vi "002_Panel01.vi"(11 "Queue Ref In":T1={"UI"=refnum, "Message"=refnum, "Data"=refnum, "Caller"=refnum, "Name"="000 Common", "Data Path"=path "", "Class Path"=path "", "SubPanel"=refnum, "Project Name"="", "MNT"="", "Title"="", "Data Source"=refnum, "Queue List"={}, "VI"=refnum, "UE"=refnum}) -> ()   [LabVIEW 2020]
uses:
  Alin/QMH/000 Module Data Type.ctl
  Alin/QMH/Queue Message.ctl
  <vilib>/Utility/file.llb/Read Delimited Spreadsheet (string).vi
  <vilib>/Utility/file.llb/Write Delimited Spreadsheet (string).vi
panel:
  in  "PanelSelect_00":u16(ring)
  in  "PanelSelect_01":u16(ring)
  in  "Panel Config":bool
  in  "Panel Refresh":bool
  in  "PanelSelect_02":u16(ring)
  in  "PanelSelect_03":u16(ring)
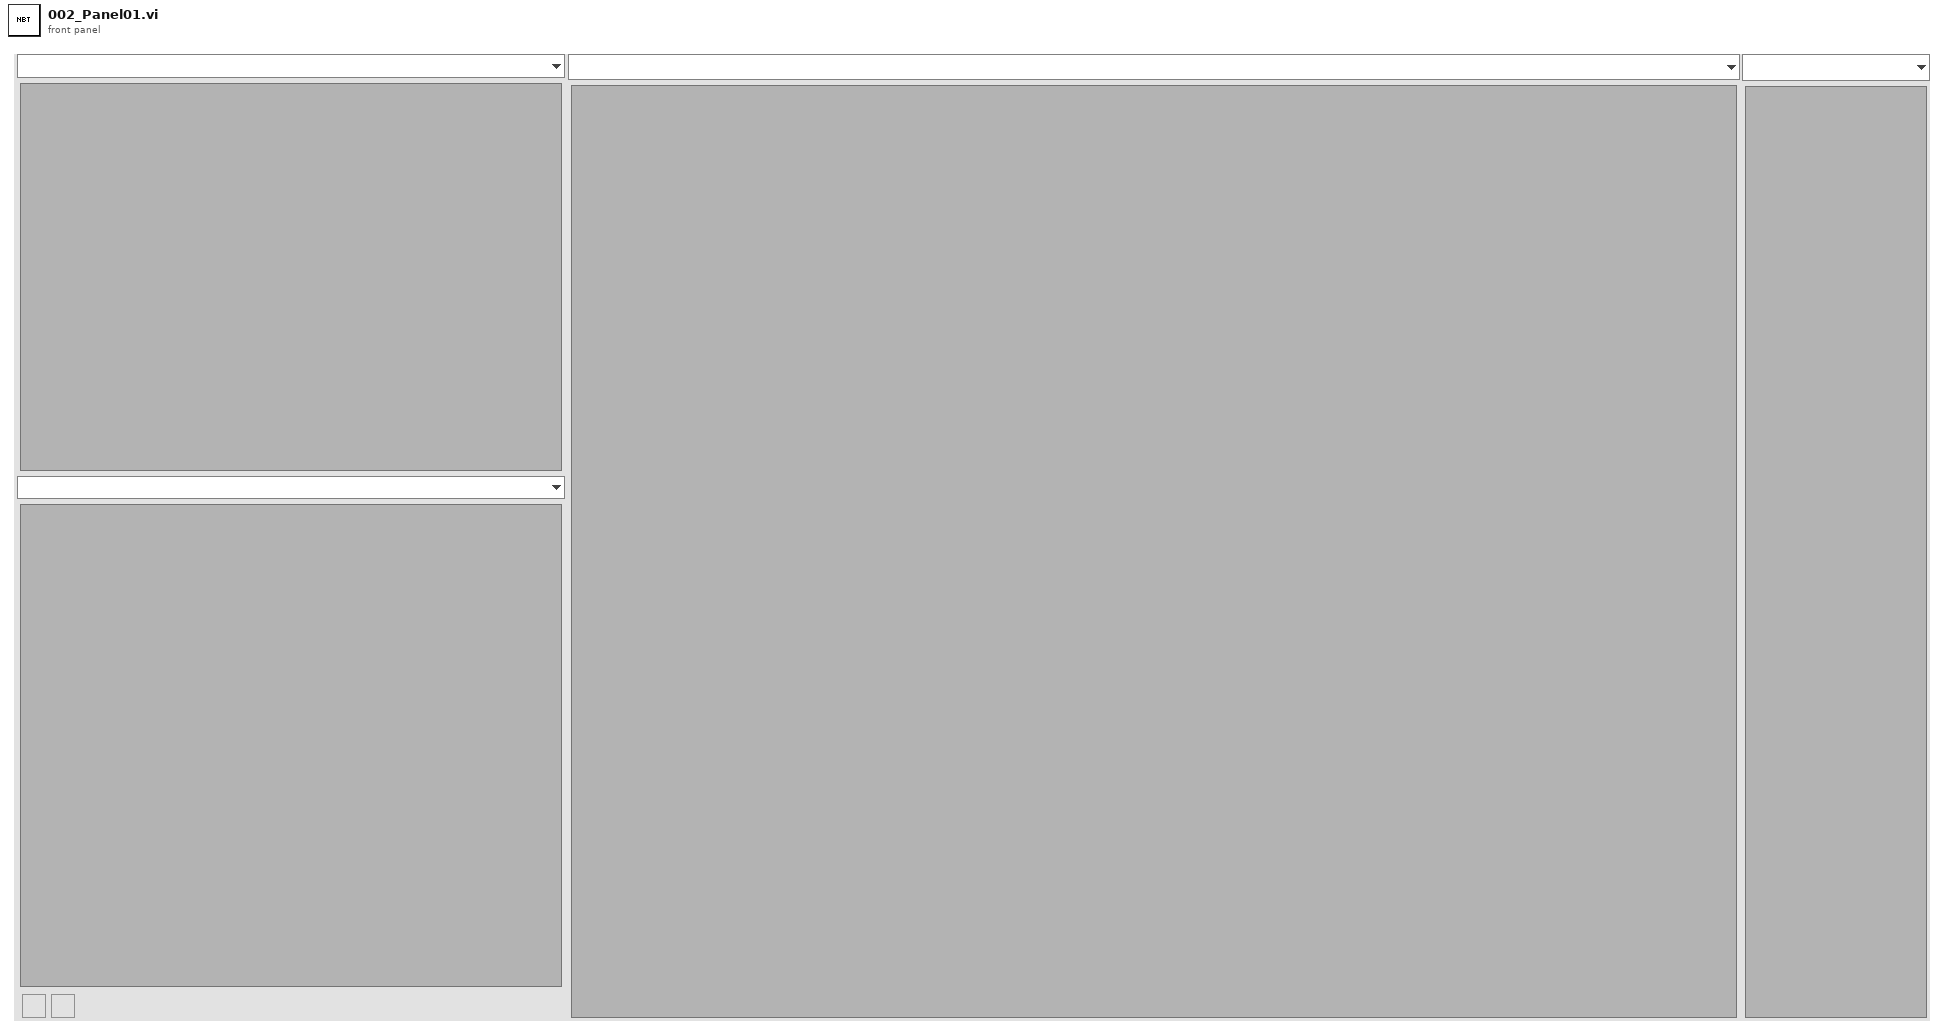
[diagram p1: front panel]
types:
  T1 = typedef "000 Module Data Type.ctl" = cluster{"UI":refnum<queue>, "Message":refnum<queue>, "Data":refnum<queue>, "Caller":refnum<queue>, "Name":string, "Data Path":path, "Class Path":path, "SubPanel":refnum<vi>, "Project Name":string, "MNT":string, "Title":string, "Data Source":refnum<queue>, "Queue List":map{string, refnum<queue>}, "VI":refnum<vi>, "UE":refnum<user-event>}
  T2 = typedef "eventvkey.ctl" = enum16{"ASCII", "Enter", "Return", "Shift", "Ctrl", "Alt", "Cmd", "Opt", "Caps", "NumLock", "Clear", "Break", "Up", "Down", "Left", "Right", "Insert", "Delete", "Home", "End", "PageUp", "PageDown", "Escape", "Help", "Pause", "ScrollLock", "F1", "F2", "F3", "F4", "F5", "F6", "F7", "F8", "F9", "F10", "F11", "F12", "F13", "F14", "F15", "F16", "F17", "F18", "F19", "F20", "F21", "F22", "F23", "F24", "Play", "VolumeUp", "VolumeDown", "Mute", "Two Byte Char"}
  T3 = cluster{"Shift":bool, "Ctrl":bool, "Alt":bool, "Cmd":bool, "Opt":bool}
  T4 = cluster{"Queue":T1, "SubPanel":cluster{"SubPanel01":refnum<vi>, "SubPanel02":refnum<vi>, "SubPanel03":refnum<vi>, "SubPanel04":refnum<vi>}, "Panel Name":string[], "PanelSelect":cluster{"PanelSelect_00":refnum<vi>, "PanelSelect_01":refnum<vi>, "PanelSelect_02":refnum<vi>, "PanelSelect_03":refnum<vi>}, "Panel Index":string[]}
  T5 = cluster{"SubPanel01":refnum<vi>, "SubPanel02":refnum<vi>, "SubPanel03":refnum<vi>, "SubPanel04":refnum<vi>}
  T6 = cluster{"PanelSelect_00":refnum<vi>, "PanelSelect_01":refnum<vi>, "PanelSelect_02":refnum<vi>, "PanelSelect_03":refnum<vi>}
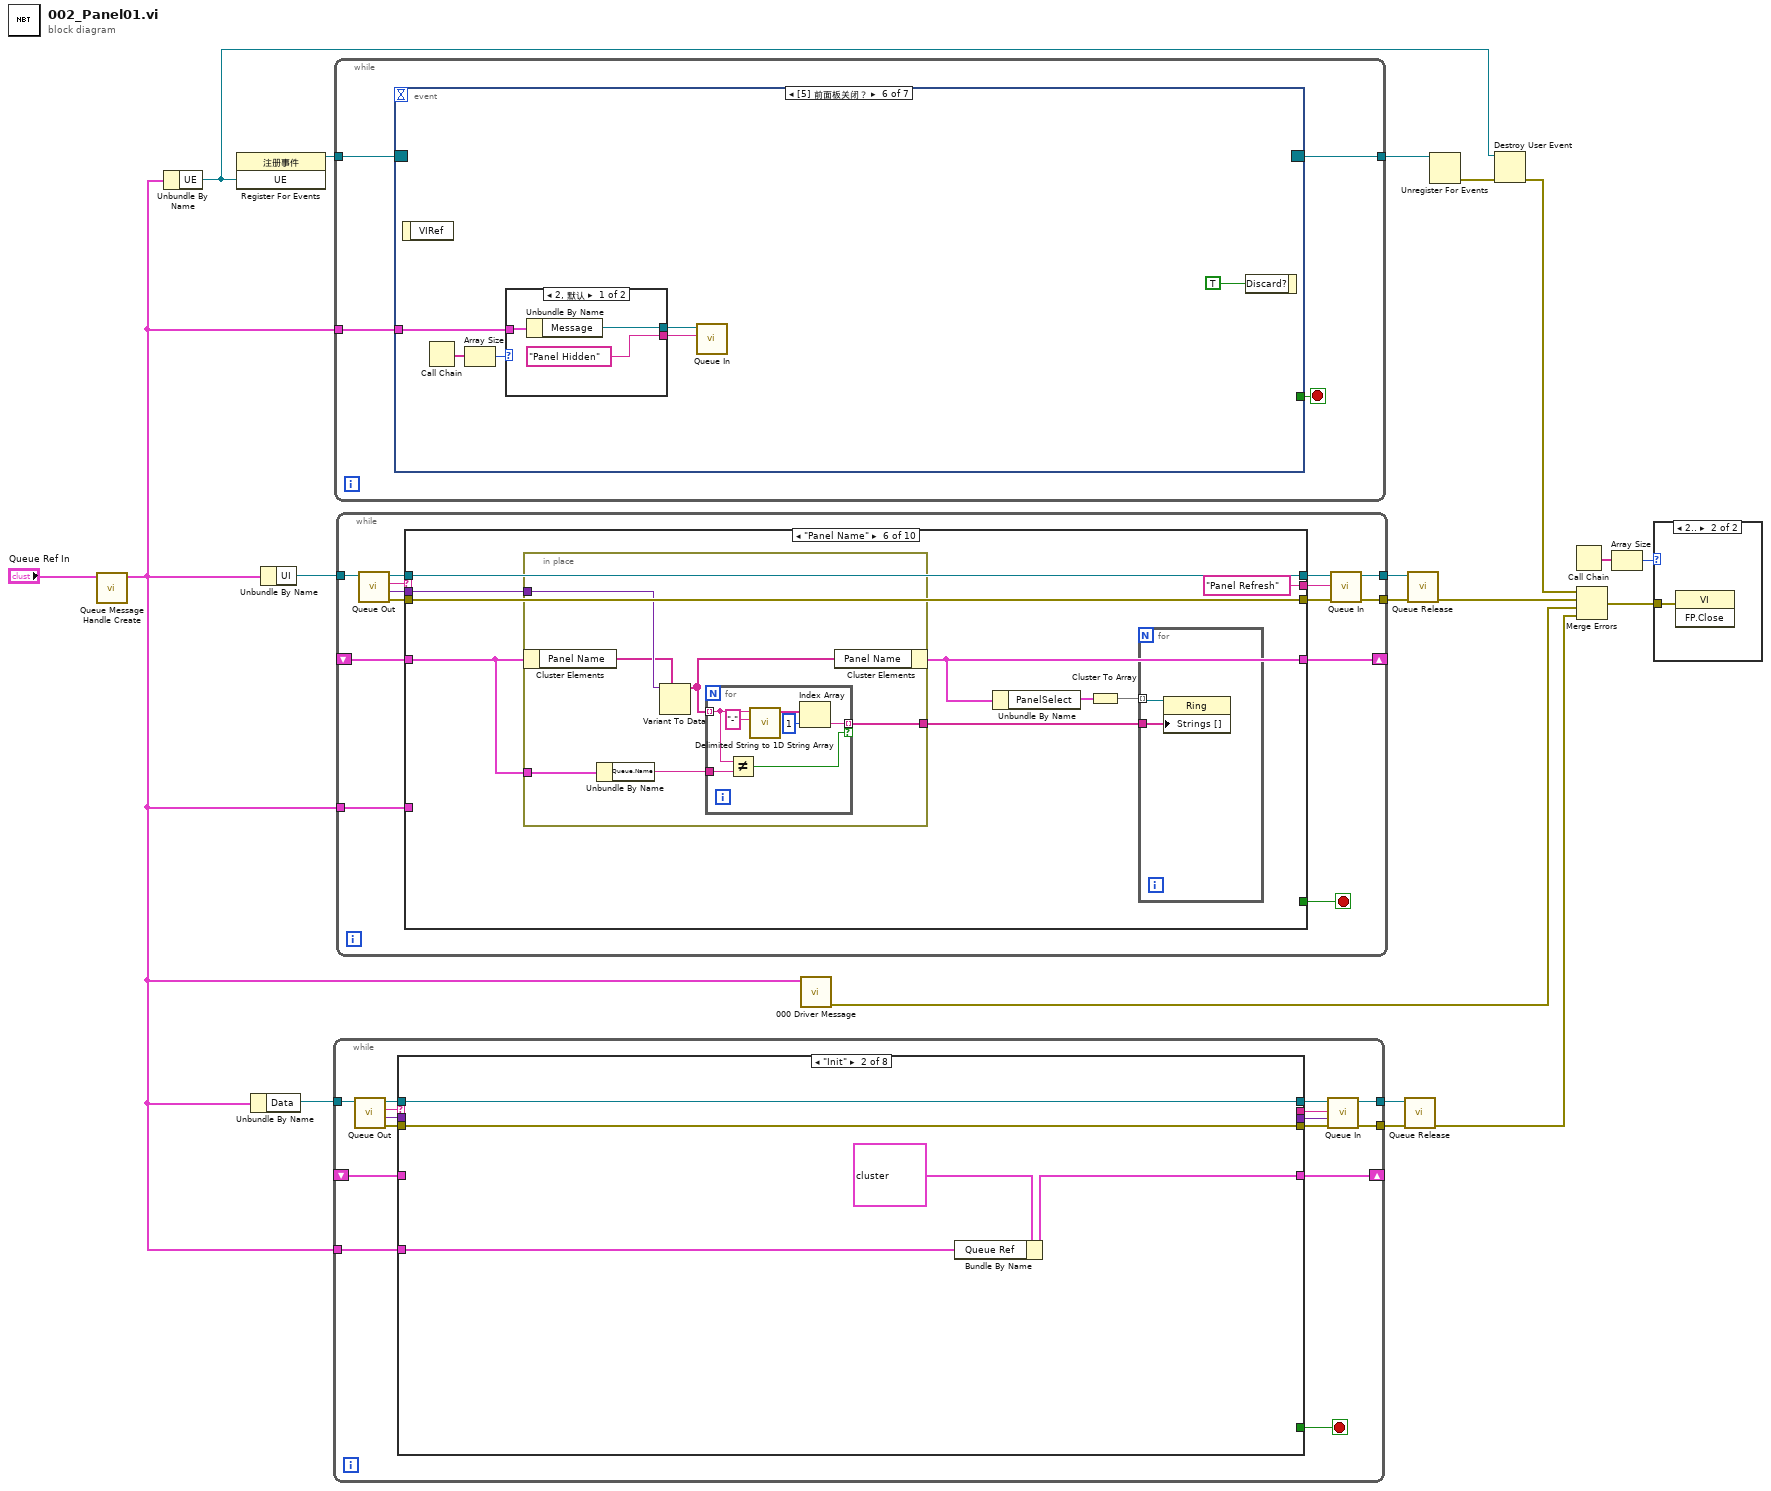
[diagram p0: block diagram]
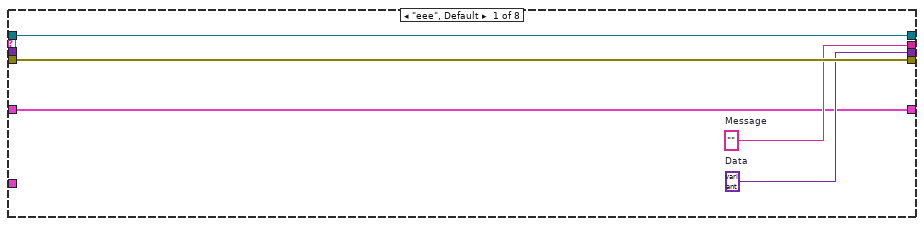
[diagram p2: hidden frame]
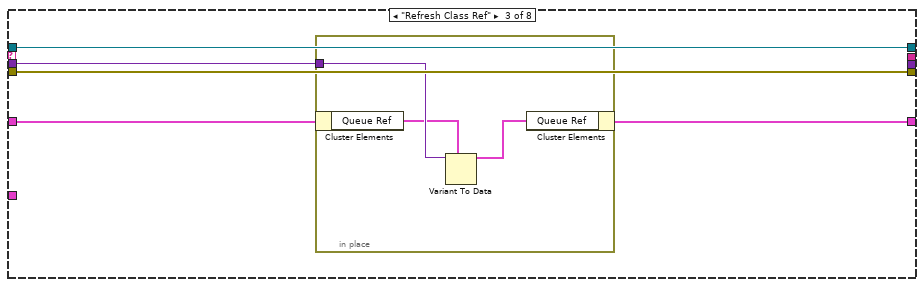
[diagram p3: hidden frame]
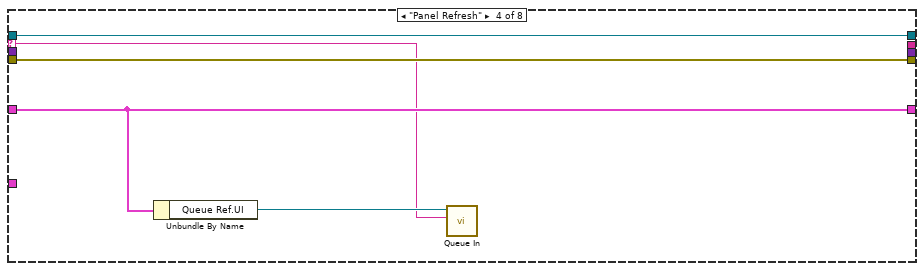
[diagram p4: hidden frame]
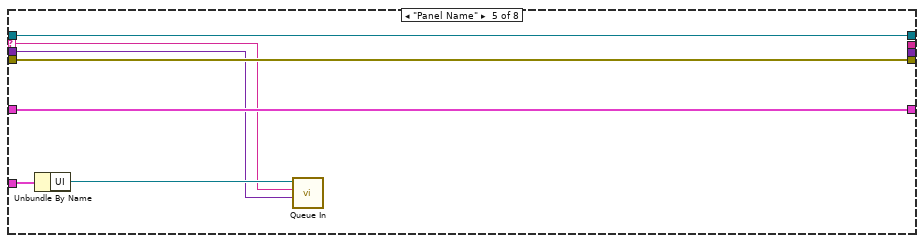
[diagram p5: hidden frame]
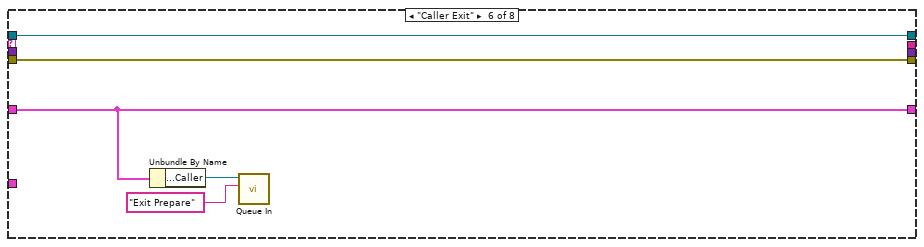
[diagram p6: hidden frame]
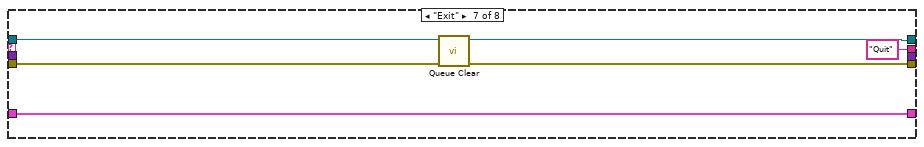
[diagram p7: hidden frame]
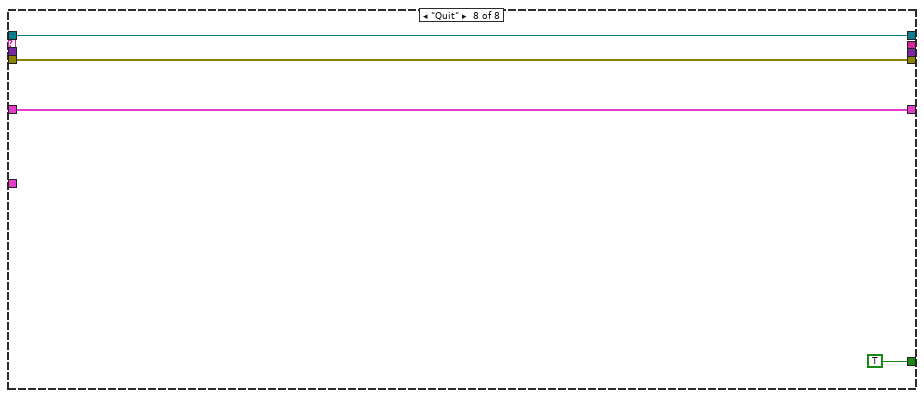
[diagram p8: hidden frame]
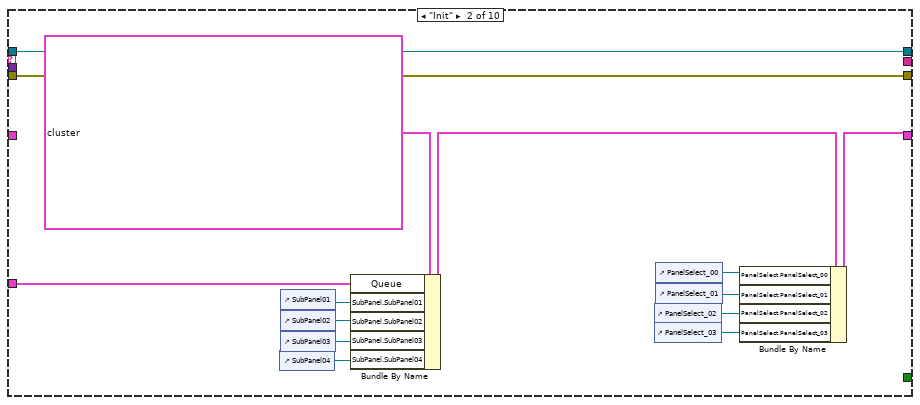
[diagram p11: hidden frame]
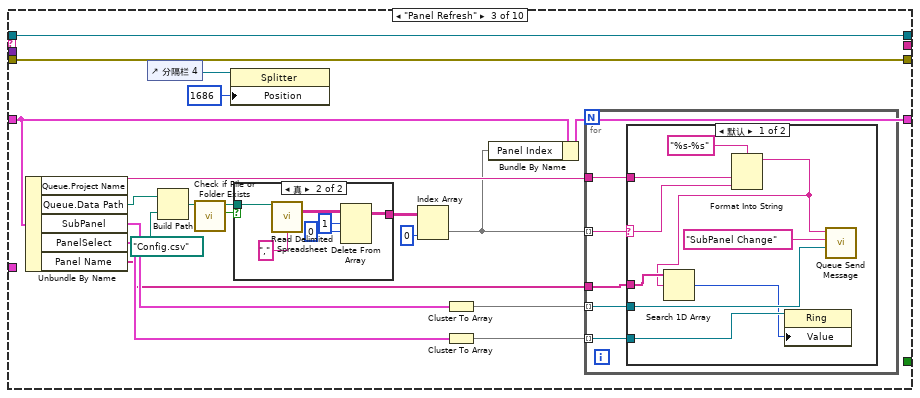
[diagram p12: hidden frame]
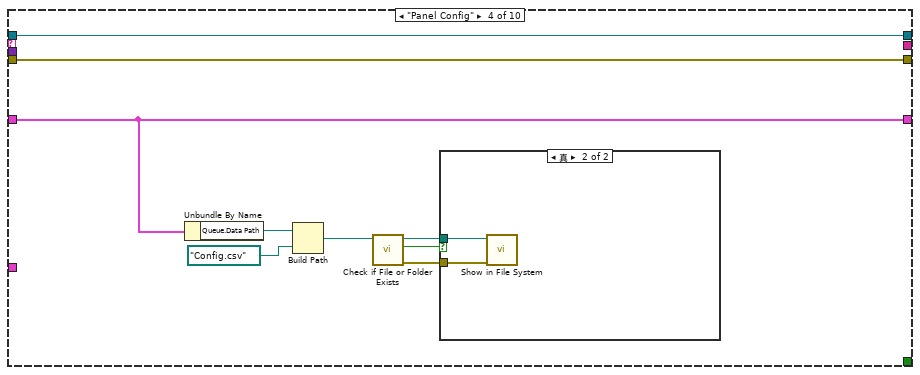
[diagram p15: hidden frame]
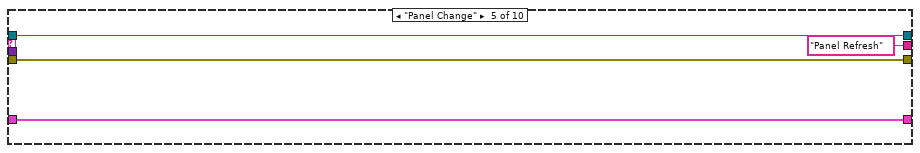
[diagram p17: hidden frame]
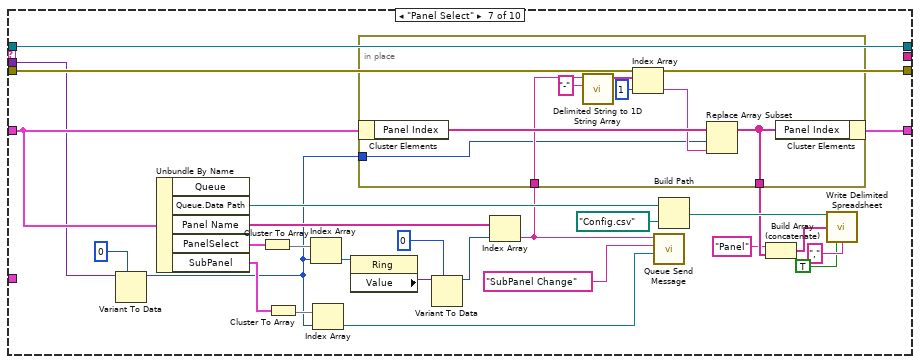
[diagram p18: hidden frame]
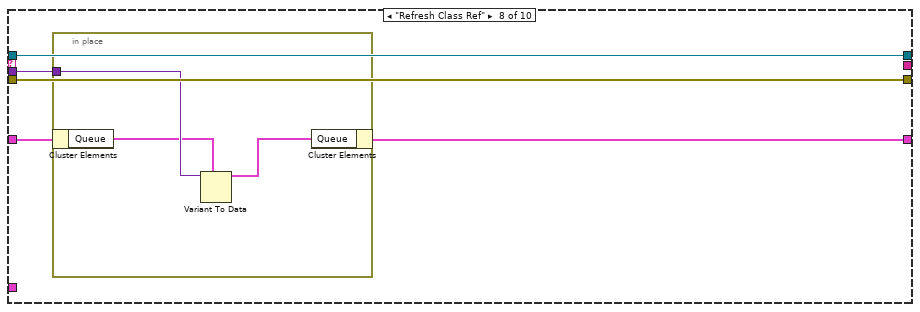
[diagram p19: hidden frame]
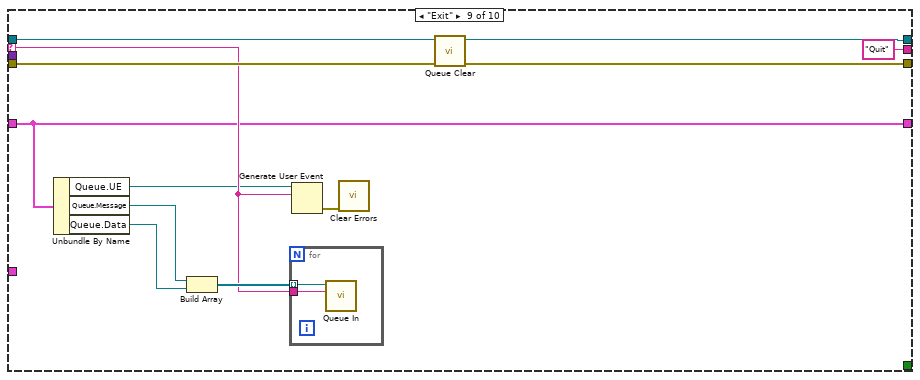
[diagram p20: hidden frame]
diagram:
  n1 = call "Queue Message Handle Create.vi"("Queue Ref In"="Queue Ref In") -> ("Queue Ref Out"=w1:T1)  [unwired: 9 in, 1 out]
  n2 = Unbundle By Name(w1) -> ("UE"=w2:refnum<user-event>)
  n3 = register-events(w2) -> (reference out=w3:refnum<event-registration>)  [unwired: 2 in, 1 out]
  n4 = Unbundle By Name(w1) -> ("Data"=w16:refnum<queue>)
  n5 = Unbundle By Name(w1) -> ("UI"=w8:refnum<queue>)
  n6 = while {
    tunnel: w16 -> [w30]
    tunnel: [w27] -> w14
    tunnel: [w26] -> w15
    shift-right: [w22] -> _
    shift-left: _ -> [w21]
    tunnel: w1 -> [w20]
    stop <- w34 stop-if-true
    n7 = call "Queue Out.vi"("Queue In"=w30) -> ("error out"=w33:errorcluster, "Data"=w31:variant, "Message"=w32:string, "Queue Out"=w29:refnum<queue>)  [unwired: 6 in, 1 out]
    n8 = case shown="\"Init\"" w32 {
      selector: w32 -> [_ _ _ w53 w59 _ _ _]
      tunnel: w29 -> [w39 w44 w49 w57 w64 w69 w74 w78]
      tunnel: w33 -> [w38 w43 w48 w56 w63 w68 w72 w79]
      tunnel: [w39 w44 w49 w57 w64 w69 w73 w78] -> w28
      tunnel: [w38 w43 w48 w56 w63 w68 w71 w79] -> w25
      tunnel: [w37 _ _ _ _ _ "Quit" _] -> w24
      tunnel: [_ _ _ _ _ _ _ TRUE] -> w34
      tunnel: [w36 _ _ _ _ _ _ _] -> w23
      tunnel: w31 -> [_ _ w45 _ w58 _ _ _]
      tunnel: [w35 w41 w46 w55 w62 w67 w70 w76] -> w22
      tunnel: w21 -> [w35 _ w47 w55 w62 w67 w70 w76]
      tunnel: w20 -> [_ w40 _ _ w61 _ _ _]
      frame "eee", Default {
        w36 = variant  # Data
        w37 = ""  # Message
      }
      frame "Init" {
        n9 = Bundle By Name(cluster=cluster{"Queue Ref ":T1} {"Queue Ref "={"UI"=refnum, "Message"=refnum, "Data"=refnum, "Caller"=refnum, "Name"="000 Common", "Data Path"=path "", "Class Path"=path "", "SubPanel"=refnum, "Project Name"="", "MNT"="", "Title"="", "Data Source"=refnum, "Queue List"={}, "VI"=refnum, "UE"=refnum}}, "Queue Ref"=w40) -> (w41:cluster{"Queue Ref ":T1})
      }
      frame "Refresh Class Ref" {
        n10 = in-place {
          in-place-border: w45 -> [w52]
          n11 = in-place-cluster #1(w47) -> ("Queue Ref"=w51:T1)
          n12 = Variant To Data(type=w51, Variant=w52) -> (data=w50:T1)  [unwired: 1 in, 1 out]
          n13 = in-place-cluster #1("Queue Ref"=w50) -> (w46:cluster{"Queue Ref ":T1})
        }
      }
      frame "Panel Refresh" {
        n14 = Unbundle By Name(w55) -> ("Queue Ref.UI"=w54:refnum<queue>)
        n15 = call "Queue In.vi"("Message"=w53, "Queue In"=w54) -> ()  [unwired: 8 in, 2 out]
      }
      frame "Panel Name" {
        n16 = Unbundle By Name(w61) -> ("UI"=w60:refnum<queue>)
        n17 = call "Queue In.vi"("Data"=w58, "Message"=w59, "Queue In"=w60) -> ()  [unwired: 7 in, 2 out]
      }
      frame "Caller Exit" {
        n18 = Unbundle By Name(w67) -> ("Queue Ref.Caller"=w66:refnum<queue>)
        n19 = call "Queue In.vi"("Message"="Exit Prepare", "Queue In"=w66) -> ()  [unwired: 8 in, 2 out]
      }
      frame "Exit" {
        n20 = call "Queue Clear.vi"("error in (no error)"=w72, "Queue In"=w74) -> ("error out"=w71:errorcluster, "Queue Out"=w73:refnum<queue>)  [unwired: 8 in]
      }
      frame "Quit" {
      }
    }
    n21 = call "Queue In.vi"("error in (no error)"=w25, "Data"=w23, "Message"=w24, "Queue In"=w28) -> ("error out"=w26:errorcluster, "Queue Out"=w27:refnum<queue>)  [unwired: 6 in]
  }
  n22 = while {
    tunnel: w3 -> [w83]
    tunnel: [w81] -> w4
    tunnel: w1 -> [w80]
    stop <- w82 stop-if-true
    n23 = event shown="[5] 前面板关闭？" {
      selector: w83 -> [_ _ _ _ _ _ _]
      dyn-events: [_ _ _ _ _ _ _] -> w81
      timeout: _ -> [_ _ _ _ _ _ _]
      tunnel: [_ _ _ _ w96 _ _] -> w82
      tunnel: w80 -> [_ w87 w91 w95 _ w99 w121]
      event Timeout {
        n24 = event-data() -> ()  [unwired: 1 in, 1 out]
      }
      event "Panel Refresh", "Panel Config": Value Change {
        n25 = event-data() -> ("CtlRef"=w85:refnum<vi>)  [unwired: 1 in]
        n26 = Unbundle By Name(w87) -> ("UI"=w86:refnum<queue>)
        n27 = property class="Bool"(reference=w85) -> ("Label.Text"=w84:string)  [unwired: 1 in, 2 out]
        n28 = call "Queue In.vi"("Message"=w84, "Queue In"=w86) -> ()  [unwired: 8 in, 2 out]
      }
      event Key Down {
        n29 = event-data() -> ("Char"=w92:i16, "VKey"=w90:T2, "Mods"=w89:cluster{"Num Pad":bool, "Menu Key":bool}, "PlatMods"=w88:T3)  [unwired: 1 in]
        n30 = call "Queue Key Down.vi"("Queue Ref Out"=w91, "C"=w92, "Platform Key"=w88, "Group Key"=w89, "V Key"=w90) -> ()  [unwired: 6 in, 1 out]
      }
      event Panel Resize; Pane Size {
        n31 = event-data() -> ()  [unwired: 1 in, 2 out]
        n32 = Unbundle By Name(w95) -> ("Data"=w94:refnum<queue>)
        n33 = call "Queue In.vi"("Message"="Panel Adjust", "Queue In"=w94) -> ()  [unwired: 8 in, 2 out]
      }
      event User Event {
        n34 = event-data() -> ("Message"=w98:string)  [unwired: 1 in]
        n35 = Equal?(x=w98, y="Exit") -> (x = y?=w96:bool)
      }
      event Panel Close? {
        n36 = event-data() -> ()  [unwired: 1 in, 1 out]
        n37 = Call Chain() -> (call chain=w103:string[])
        n38 = Array Size(array=w103) -> (size(s)=w102:i32)
        n39 = case shown="2, 默认" w102 {
          tunnel: w99 -> [w107 w110]
          tunnel: [w106 w109] -> w101
          tunnel: ["Panel Hidden" ("Message") "Exit Prepare" ("Message")] -> w100
          frame 2, Default {
            n40 = Unbundle By Name(w107) -> ("Message"=w106:refnum<queue>)
          }
          frame 1 {
            n41 = Unbundle By Name(w110) -> ("Message"=w109:refnum<queue>)
          }
        }
        n42 = call "Queue In.vi"("Message"=w100, "Queue In"=w101) -> ()  [unwired: 8 in, 2 out]
        n43 = event-data("Discard?"=TRUE ("放弃？")) -> ()  [unwired: 1 in, 1 out]
      }
      event "PanelSelect_01", "PanelSelect_00", "PanelSelect_02", "PanelSelect_03": Value Change {
        n44 = event-data() -> ("CtlRef"=w118:refnum<vi>)  [unwired: 1 in]
        n45 = Unbundle By Name(w121) -> ("UI"=w120:refnum<queue>)
        n46 = property class="Ring (严格)"(reference=w118) -> ("Label.Text"=w117:string)  [unwired: 1 in, 2 out]
        n47 = call <vilib>:"Delimited String to 1D String Array.vi"("delimiter"="_", "delimited string"=w117) -> ("string array"=w115:string[])  [unwired: 9 in]
        n48 = Index Array(array=w115, index=1 ("索引")) -> (element=w113:string)
        n49 = Fract/Exp String To Number(string=w113, default (0 dbl)=u32 0 ("默认(0 DBL)")) -> (number=w111:u32)  [unwired: 2 in, 1 out]
        n50 = call "Queue In.vi"("Data"=w111, "Message"="Panel Select", "Queue In"=w120) -> ()  [unwired: 7 in, 2 out]
      }
    }
  }
  n51 = while {
    tunnel: w8 -> [w131]
    tunnel: [w128] -> w6
    tunnel: [w127] -> w7
    shift-right: [w124] -> _
    shift-left: _ -> [w123]
    tunnel: w1 -> [w122]
    stop <- w135 stop-if-true
    n52 = call "Queue Out.vi"("Queue In"=w131) -> ("error out"=w134:errorcluster, "Data"=w132:variant, "Message"=w133:string, "Queue Out"=w130:refnum<queue>)  [unwired: 6 in, 1 out]
    n53 = case shown="\"Panel Name\"" w133 {
      selector: w133 -> [_ _ _ _ _ _ _ _ w280 _]
      tunnel: w130 -> [w138 w152 w172 w201 w207 w216 w258 w271 w285 w291]
      tunnel: w134 -> [w137 w151 w171 w200 w206 w215 w257 w270 w283 w292]
      tunnel: [w138 w152 w172 w201 w207 w216 w258 w271 w284 w291] -> w129
      tunnel: [w137 w151 w171 w200 w206 w215 w257 w270 w282 w292] -> w126
      tunnel: [_ _ _ _ "Panel Refresh" "Panel Refresh" _ _ "Quit" _] -> w125
      tunnel: [_ _ _ _ _ _ _ _ _ TRUE] -> w135
      tunnel: w132 -> [_ _ _ _ _ w214 w253 w268 _ _]
      tunnel: [w136 w143 w157 w198 w205 w213 w240 w267 w278 w289] -> w124
      tunnel: w123 -> [w136 _ w170 w198 w205 w208 w256 w269 w278 w289]
      tunnel: w122 -> [_ w148 _ _ _ _ _ _ _ _]
      frame "eee", Default {
      }
      frame "Init" {
        n54 = control-ref of="SubPanel04"() -> (w144:refnum<vi>)
        n55 = control-ref of="SubPanel01"() -> (w145:refnum<vi>)
        n56 = control-ref of="SubPanel02"() -> (w146:refnum<vi>)
        n57 = control-ref of="SubPanel03"() -> (w147:refnum<vi>)
        n58 = Bundle By Name(cluster=T4 {"Queue"={"UI"=refnum, "Message"=refnum, "Data"=refnum, "Caller"=refnum, "Name"="000 Common", "Data Path"=path "", "Class Path"=path "", "SubPanel"=refnum, "Project Name"="", "MNT"="", "Title"="", "Data Source"=refnum, "Queue List"={}, "VI"=refnum, "UE"=refnum}, "SubPanel"={"SubPanel01"=refnum, "SubPanel02"=refnum, "SubPanel03"=refnum, "SubPanel04"=refnum}, "Panel Name"=[], "PanelSelect"={"PanelSelect_00"=refnum, "PanelSelect_01"=refnum, "PanelSelect_02"=refnum, "PanelSelect_03"=refnum}, "Panel Index"=[]}, "Queue"=w148, "SubPanel.SubPanel01"=w145, "SubPanel.SubPanel02"=w146, "SubPanel.SubPanel03"=w147, "SubPanel.SubPanel04"=w144) -> (w149:T4)
        n59 = control-ref of="PanelSelect_02"() -> (w142:refnum<vi>)
        n60 = control-ref of="PanelSelect_03"() -> (w141:refnum<vi>)
        n61 = control-ref of="PanelSelect_00"() -> (w139:refnum<vi>)
        n62 = control-ref of="PanelSelect_01"() -> (w140:refnum<vi>)
        n63 = Bundle By Name(cluster=w149, "PanelSelect.PanelSelect_00"=w139, "PanelSelect.PanelSelect_01"=w140, "PanelSelect.PanelSelect_02"=w142, "PanelSelect.PanelSelect_03"=w141) -> (w143:T4)
      }
      frame "Panel Refresh" {
        n64 = Unbundle By Name(w170) -> ("Queue.Project Name"=w160:string, "Queue.Data Path"=w163:path, "SubPanel"=w165:T5, "PanelSelect"=w155:T6, "Panel Name"=w153:string[])
        n65 = control-ref of="分隔栏 4"() -> (w159:refnum<vi>)
        n66 = Build Path(base path=w163, name or relative path=path "Config.csv" ("名称或相对路径")) -> (appended path=w161:path)
        n67 = call <vilib>:"Check if File or Folder Exists.vi"("path"=w161) -> ("file or folder exists?"=w168:bool, "dup path"=w169:path)  [unwired: 8 in, 1 out]
        n68 = property class="Splitter"(reference=w159, "Position"=1686 ("分隔栏位置")) -> ()  [unwired: 1 in, 2 out]
        n69 = case shown="真" w168 {
          tunnel: w169 -> [_ w191]
          tunnel: [_ w187] -> w167
          frame False {
          }
          frame True {
            n70 = call-poly <vilib>:"Read Delimited Spreadsheet.vi"("file path (dialog if empty)"=w191, "delimiter (\\t)"="," ("delimiter (\\t)")) -> ("all rows"=w190:string[][])  [unwired: 8 in, 5 out]
            n71 = Delete From Array(array=w190, length=1 ("长度"), index (row)=0 ("索引 (行)")) -> (array with subset deleted=w187:string[][])  [unwired: 1 in, 1 out]
          }
        }
        n72 = Index Array(array=w167, index (col)=0 ("禁用的索引 (列)")) -> (element=w156:string[])  [unwired: 1 in]
        n73 = Cluster To Array(cluster=w165) -> (array=w164:refnum<vi>[])
        n74 = Cluster To Array(cluster=w155) -> (array=w154:refnum<vi>[])
        n75 = Bundle By Name(cluster=w170, "Panel Index"=w156) -> (w157:T4)
        n76 = for {
          tunnel: w156 -> [w175] mode=indexing
          tunnel: w164 -> [w177] mode=indexing
          tunnel: w160 -> [w176]
          tunnel: w154 -> [w174] mode=indexing
          tunnel: w153 -> [w173]
          n77 = case shown="默认" w175 {
            selector: w175 -> [w183 _]
            tunnel: w177 -> [w185 _]
            tunnel: w176 -> [w180 _]
            tunnel: w174 -> [w182 _]
            tunnel: w173 -> [w181 _]
            frame Default {
              n78 = Format Into String(format string="%s-%s" ("格式字符串"), w180, w183) -> (resulting string=w178:string)  [unwired: 2 in, 1 out]
              n79 = Search 1D Array(1D array=w181, element=w178) -> (index of element=w179:i32)  [unwired: 1 in]
              n80 = property class="Ring"(reference=w182, "Value"=w179) -> ()  [unwired: 1 in, 2 out]
              n81 = call "Queue Send Message.vi"("Data"=w185, "Message"="SubPanel Change", "Queue Name"=w178) -> ()  [unwired: 6 in, 3 out]
            }
            frame "" {
            }
          }
        }
      }
      frame "Panel Config" {
        n82 = Unbundle By Name(w198) -> ("Queue.Data Path"=w197:path)
        n83 = Build Path(base path=w197, name or relative path=path "Config.csv" ("名称或相对路径")) -> (appended path=w196:path)
        n84 = call <vilib>:"Check if File or Folder Exists.vi"("path"=w196) -> ("error out"=w193:errorcluster, "file or folder exists?"=w195:bool, "dup path"=w194:path)  [unwired: 8 in]
        n85 = case shown="真" w195 {
          tunnel: w194 -> [_ w203]
          tunnel: w193 -> [_ w202]
          frame False {
          }
          frame True {
            n86 = call <vilib>:"Show in File System.vi"("error in (no error)"=w202, "file or directory path"=w203) -> ()  [unwired: 9 in, 1 out]
          }
        }
      }
      frame "Panel Change" {
      }
      frame "Panel Name" {
        n87 = in-place {
          in-place-border: w214 -> [w224]
          in-place-border: [w221] -> w210
          in-place-border: w208 -> [w220]
          n88 = in-place-cluster #2(w208) -> ("Panel Name"=w223:string[])
          n89 = Unbundle By Name(w220) -> ("Queue.Name"=w219:string)
          n90 = Variant To Data(type=w223, Variant=w224) -> (data=w222:string[])  [unwired: 1 in, 1 out]
          n91 = for {
            tunnel: w222 -> [w227] mode=indexing
            tunnel: [w228] -> w221 mode=indexing if=w225
            tunnel: w219 -> [w226]
            n92 = Not Equal?(x=w227, y=w226) -> (x != y?=w225:bool)
            n93 = call <vilib>:"Delimited String to 1D String Array.vi"("delimiter"="-", "delimited string"=w227) -> ("string array"=w230:string[])  [unwired: 9 in]
            n94 = Index Array(array=w230, index=1 ("索引")) -> (element=w228:string)
          }
          n95 = in-place-cluster #2("Panel Name"=w222) -> (w213:T4)
        }
        n96 = Unbundle By Name(w213) -> ("PanelSelect"=w212:T6)
        n97 = Cluster To Array(cluster=w212) -> (array=w211:refnum<vi>[])
        n98 = for {
          tunnel: w211 -> [w218] mode=indexing
          tunnel: w210 -> [w217]
          n99 = property class="Ring"(reference=w218, "Strings []"=w217) -> ()  [unwired: 1 in, 2 out]
        }
      }
      frame "Panel Select" {
        n100 = Variant To Data(type=u32 0 ("数字"), Variant=w253) -> (data=w232:u32)  [unwired: 1 in, 1 out]
        n101 = Unbundle By Name(w256) -> ("Queue.Data Path"=w243:path, "Panel Name"=w255:string[], "PanelSelect"=w251:T6, "SubPanel"=w245:T5)  [unwired: 1 out]
        n102 = Cluster To Array(cluster=w251) -> (array=w250:refnum<vi>[])
        n103 = Cluster To Array(cluster=w245) -> (array=w246:refnum<vi>[])
        n104 = Index Array(array=w250, index=w232) -> (element=w249:refnum<vi>)
        n105 = Index Array(array=w246, index=w232) -> (element=w244:refnum<vi>)
        n106 = property class="Ring"(reference=w249) -> ("Value"=w248:variant)  [unwired: 1 in, 2 out]
        n107 = Variant To Data(type=u16 0 ("PanelSelect_03"), Variant=w248) -> (data=w239:u16)  [unwired: 1 in, 1 out]
        n108 = Index Array(array=w255, index=w239) -> (element=w238:string)
        n109 = in-place {
          in-place-border: w238 -> [w262]
          in-place-border: [w260] -> w236
          in-place-border: w232 -> [w259]
          n110 = in-place-cluster #3(w256) -> ("Panel Index"=w266:string[])
          n111 = call <vilib>:"Delimited String to 1D String Array.vi"("delimiter"="-", "delimited string"=w262) -> ("string array"=w264:string[])  [unwired: 9 in]
          n112 = Index Array(array=w264, index=1 ("索引")) -> (element=w261:string)
          n113 = Replace Array Subset(array=w266, new element=w261, index=w259) -> (w260:string[])
          n114 = in-place-cluster #3("Panel Index"=w260) -> (w240:T4)
        }
        n115 = call "Queue Send Message.vi"("Data"=w244, "Message"="SubPanel Change", "Queue Name"=w238) -> ()  [unwired: 6 in, 3 out]
        n116 = Build Path(base path=w243, name or relative path=path "Config.csv" ("名称或相对路径")) -> (appended path=w241:path)
        n117 = Build Array (concatenate)("Panel", w236) -> (w235:string[])
        n118 = call-poly <vilib>:"Write Delimited Spreadsheet.vi"("file path (dialog if empty)"=w241, "1D data"=w235, "transpose? (no:F)"=TRUE, "delimiter (\\t)"="," ("delimiter (\\t)")) -> ()  [unwired: 10 in, 2 out]
      }
      frame "Refresh Class Ref" {
        n119 = in-place {
          in-place-border: w268 -> [w274]
          n120 = in-place-cluster #4(w269) -> ("Queue"=w273:T1)
          n121 = Variant To Data(type=w273, Variant=w274) -> (data=w272:T1)  [unwired: 1 in, 1 out]
          n122 = in-place-cluster #4("Queue"=w272) -> (w267:T4)
        }
      }
      frame "Exit" {
        n123 = Unbundle By Name(w278) -> ("Queue.UE"=w277:refnum<user-event>, "Queue.Message"=w276:refnum<queue>, "Queue.Data"=w275:refnum<queue>)
        n124 = Build Array(w276, w275) -> (w281:refnum<queue>[])
        n125 = for {
          tunnel: w281 -> [w288] mode=indexing
          tunnel: w280 -> [w287]
          n126 = call "Queue In.vi"("Message"=w287, "Queue In"=w288) -> ()  [unwired: 8 in, 2 out]
        }
        n127 = Generate User Event(user event=w277, event data cluster=w280) -> (error out=w279:errorcluster)  [unwired: 2 in, 1 out]
        n128 = call <vilib>:"Clear Errors.vi"("error in (no error)"=w279) -> ()  [unwired: 5 in, 2 out]
        n129 = call "Queue Clear.vi"("error in (no error)"=w283, "Queue In"=w285) -> ("error out"=w282:errorcluster, "Queue Out"=w284:refnum<queue>)  [unwired: 8 in]
      }
      frame "Quit" {
      }
    }
    n130 = call "Queue In.vi"("error in (no error)"=w126, "Message"=w125, "Queue In"=w129) -> ("error out"=w127:errorcluster, "Queue Out"=w128:refnum<queue>)  [unwired: 7 in]
  }
  n131 = call "000 Driver Message.vi"("Queue In"=w1) -> ("error out"=w18:errorcluster)  [unwired: 8 in, 2 out]
  n132 = call "Queue Release.vi"("error in (no error)"=w15, "Queue In"=w14) -> ("error out"=w17:errorcluster)  [unwired: 9 in]
  n133 = call "Queue Release.vi"("error in (no error)"=w7, "Queue In"=w6) -> ("error out"=w10:errorcluster)  [unwired: 9 in]
  n134 = Unregister For Events(event registration refnum=w4) -> (error out=w5:errorcluster)  [unwired: 1 in]
  n135 = Destroy User Event(user event=w2, error in=w5) -> (error out=w9:errorcluster)
  n136 = Call Chain() -> (call chain=w12:string[])
  n137 = Merge Errors(w9, w10, w18, w17) -> (w11:errorcluster)
  n138 = Array Size(array=w12) -> (size(s)=w13:i32)
  n139 = case shown="2.." w13 {
    tunnel: w11 -> [_ w293]
    frame 0, Default {
    }
    frame 2.. {
      n140 = invoke class="VI" method="FP.Close"(error in=w293) -> ()  [unwired: 2 in, 3 out]
    }
  }
